vi "String Event Test.vi"() -> ()   [LabVIEW 2017]
uses:
  <vilib>/Utility/miscctls.llb/LVSelectionTypeDef.ctl
  <vilib>/Utility/miscctls.llb/LVFontTypeDef.ctl
panel:
  out "Text.Font":T1
  out "Text.Font:Size":u32
  out "Text.Size:Height":u32
  out "Size:Height":u32
  out "Text.Selection":T2
  out "Text.Scroll Position":u32
  in  "stop":bool
  in  "channel count":i32=100
  out "Values":string
  out "ASCII":string
  out "Hex":string
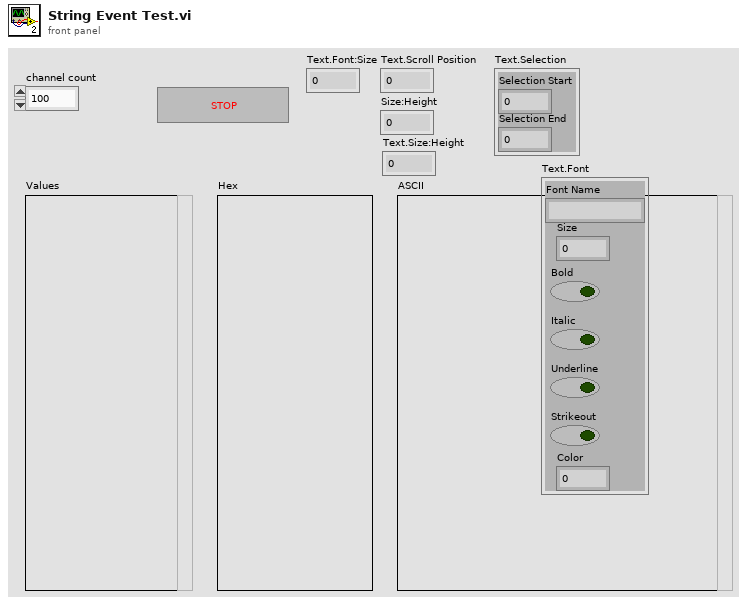
[diagram p1: front panel]
types:
  T1 = typedef "LVFontTypeDef.ctl" = cluster{"Font Name":string, "Size":u16, "Bold":bool, "Italic":bool, "Underline":bool, "Strikeout":bool, "Color":u32}
  T2 = typedef "LVSelectionTypeDef.ctl" = cluster{"Selection Start":u32, "Selection End":u32}
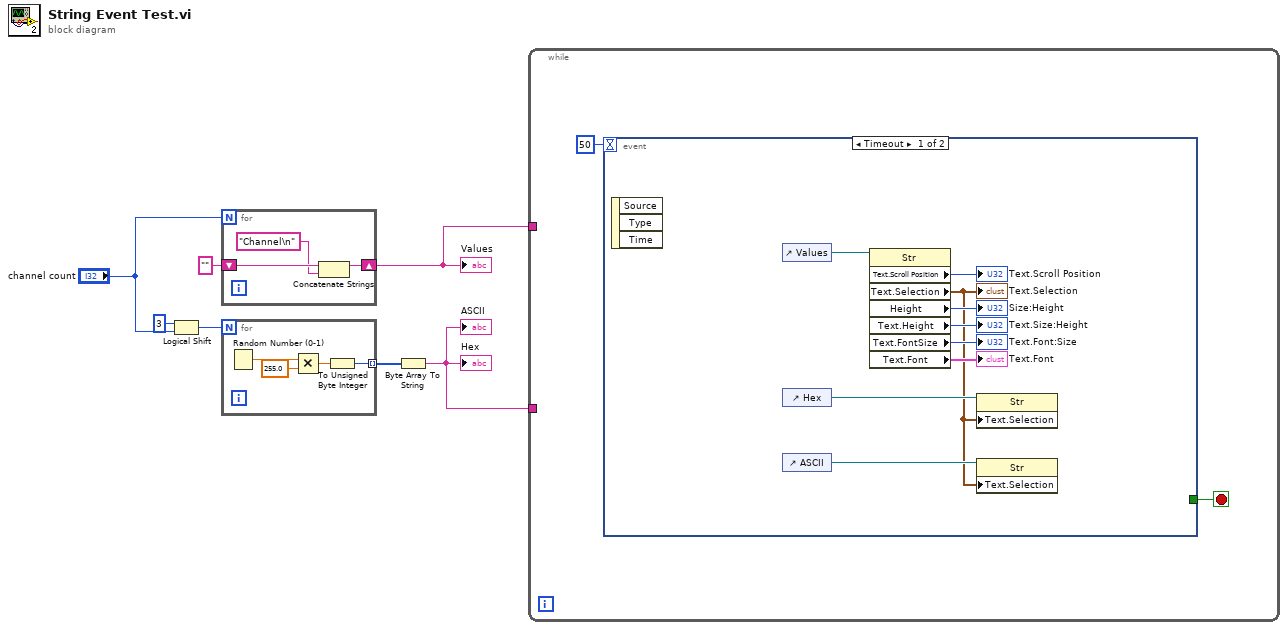
[diagram p0: block diagram]
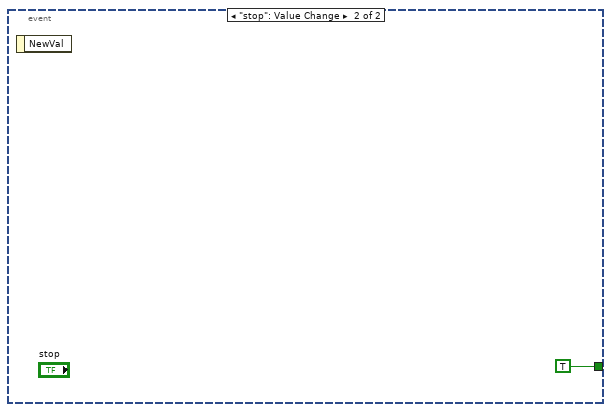
[diagram p2: hidden frame]
diagram:
  n1 = Logical Shift(y=i16 3, x="channel count") -> (x << y=w5:i32)
  n2 = for {
    N: "channel count" -> [_]
    shift-right: [w10] -> w2
    shift-left: "" -> [w9]
    n3 = Concatenate Strings(w9, "Channel\n") -> (w10:string)
  }
  "Values" <- w2
  n4 = for {
    N: w5 -> [_]
    tunnel: [w11] -> w7 mode=indexing
    n5 = Random Number (0-1)() -> (number: 0 to 1=w14:dbl)
    n6 = Multiply(x=w14, y=255.0) -> (x*y=w12:dbl)
    n7 = To Unsigned Byte Integer(number=w12) -> (unsigned 8bit integer=w11:u8)
  }
  n8 = Byte Array To String(unsigned byte array=w7) -> (string=w1:string)
  "Hex" <- w1
  "ASCII" <- w1
  n9 = while {
    tunnel: w2 -> [_]
    tunnel: w1 -> [_]
    stop <- w16 stop-if-true
    n10 = event shown="[0] Timeout" {
      selector: _ -> [_ _]
      dyn-events: _ -> [_ _]
      timeout: 50 -> [_ _]
      tunnel: [_ TRUE] -> w16
      event Timeout {
        n11 = event-data() -> ()  [unwired: 1 in, 3 out]
        n12 = control-ref of="Values"() -> (w25:refnum<vi>)
        n13 = control-ref of="Hex"() -> (w22:refnum<vi>)
        n14 = control-ref of="ASCII"() -> (w24:refnum<vi>)
        n15 = property class="Str"(reference=w25) -> ("Text.Scroll Position"=→"Text.Scroll Position":u32, "Text.Selection"=w17:T2, "Height"=→"Size:Height":u32, "Text.Height"=→"Text.Size:Height":u32, "Text.FontSize"=→"Text.Font:Size":u32, "Text.Font"=→"Text.Font":T1)  [unwired: 1 in, 2 out]
        "Text.Selection" <- w17
        n16 = property class="Str"(reference=w22, "Text.Selection"=w17) -> ()  [unwired: 1 in, 2 out]
        n17 = property class="Str"(reference=w24, "Text.Selection"=w17) -> ()  [unwired: 1 in, 2 out]
      }
      event "stop": Value Change {
        n18 = event-data() -> ()  [unwired: 1 in, 1 out]
      }
    }
  }
